vi "CONEX-ALL Reset Controller's Address To 1 v2.vi"(9 "Connection Cluster in":T1) -> (3 "Connection Cluster out":T1)   [LabVIEW 2010]
doc: "RS## - Reset controller's address to 1\n\nNo parameters in or out.\n\nA 3 second delay is there to verify address has been changed before next command, and address is changed to 1 in Connection cluster."
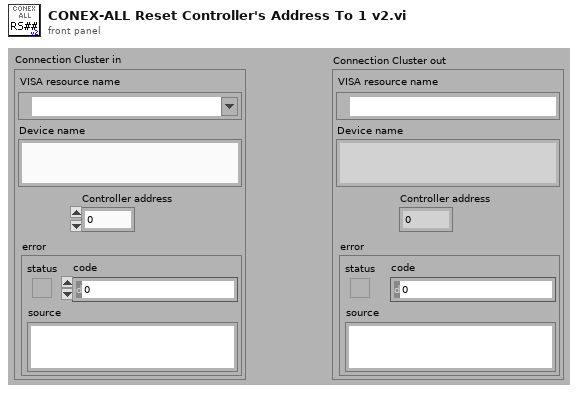
[diagram p1: front panel]
types:
  T1 = cluster{"VISA resource name":refnum<visa-resource-name>, "Device name":string, "Controller address":i32, "error":errorcluster}
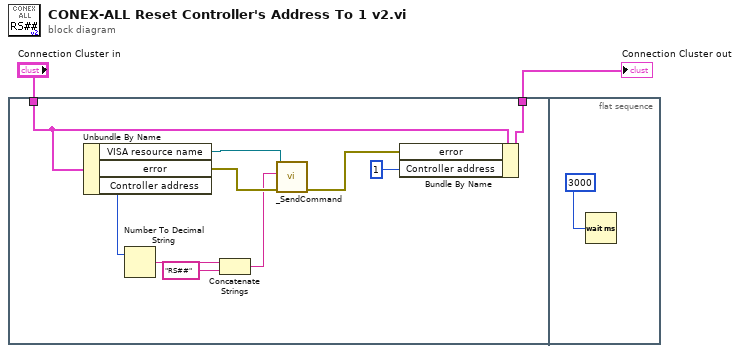
[diagram p0: block diagram]
diagram:
  n1 = flat-sequence {
    tunnel: "Connection Cluster in" -> [w7]
    tunnel: [w6] -> w1
    frame #0 {
      n2 = Unbundle By Name(w7) -> ("VISA resource name"=w10:refnum<visa-resource-name>, "error"=w8:errorcluster, "Controller address"=w5:i32)
      n3 = Number To Decimal String(number=w5) -> (decimal integer string=w12:string)  [unwired: 1 out]
      n4 = Concatenate Strings(w12, "RS##" ("strCommand")) -> (w4:string)
      n5 = call <userlib>:"_SendCommand.vi"("error in"=w8, "Command"=w4, "Instrument Channel"=w10) -> ("error out"=w9:errorcluster)  [unwired: 7 in, 1 out]
      n6 = Bundle By Name(cluster=w7, "error"=w9, "Controller address"=1) -> (w6:T1)
    }
    frame #1 {
      n7 = Wait (ms)(milliseconds to wait=3000) -> ()  [unwired: 1 out]
    }
  }
  "Connection Cluster out" <- w1
